vi "Subvi trigger AO DO.vi"(9 "Ext trig enable":bool) -> ()   [LabVIEW 2017]
uses:
  <vilib>/Platform/TimedLoop/XDataNode/timing_clust.ctl
  <vilib>/Platform/TimedLoop/XDataNode/nitl_modes.ctl
  <vilib>/Platform/TimedLoop/XDataNode/wakeup.ctl
  <vilib>/rvi/Emulation/niFpgaSctlEmulationGetInTimedLoop.vi
  <vilib>/rvi/Emulation/niFpgaEmulationReportErrorSimple.vi
  <vilib>/rvi/Emulation/niFpgaGetClockAttributes.vi
  <vilib>/rvi/Emulation/niFpgaCriticalErrorInLSC.vi
  Detector/GV subtrigger.vi
  GV trigger delay.vi
  <vilib>/Platform/TimedLoop/XDataNode/XDataNode.xnode
  <vilib>/Platform/TimedLoop/XDataNode/XDNodeRunTimeDep.lvlib
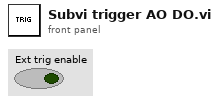
[diagram p1: front panel]
types:
  T1 = typedef "XDNodeRunTimeDep.lvlib/timing_clust.ctl" = cluster{"Expected End [f-1]":u64, "Actual End [f-1]":u64, "Finished Late? [f-1]":bool, "Expected End [i-1]":u64, "Actual End [i-1]":u64, "Finished Late? [i-1]":bool, "Expected Start [i]":u64, "Actual Start [i]":u64, "Expected Start [f]":u64, "Actual Start [f]":u64, "Source Name":string, "Structure Name":string, "Period":i64, "Deadline":i64, "Offset":i64, "Start":i64, "Priority":i32, "Timeout":i32, "Mode":T2, "Wakeup Reason":T3, "Error":errorcluster, "Source Type":string, "Secondary Source Type":string, "Global End Time":u64, "Global Start Time":u64, "Frame Duration":u64, "Iteration Duration":u64, "Assigned CPU":i32, "I/O Scan Engine Mode":u32}
  T2 = typedef "XDNodeRunTimeDep.lvlib/nitl_modes.ctl" = enum32{"No Change", "Process missed periods, maintain original phase", "Discard missed periods, maintain original phase", "Process missed periods, ignore original phase", "Discard missed periods, ignore original phase"}
  T3 = typedef "XDNodeRunTimeDep.lvlib/wakeup.ctl" = enum32{"Normal", "Aborted", "Asynchronous wakeup", "Timing source error", "Timed loop error", "Timeout"}
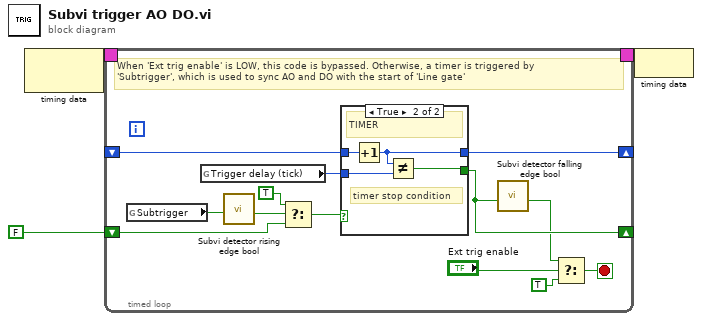
[diagram p0: block diagram]
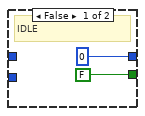
[diagram p2: hidden frame]
diagram:
  n1 = node-c288() -> (w3:T1)  [unwired: 1 in]
  n2 = timed-loop {
    timing: w3 -> [_]
    timing-out: [_] -> w2
    shift-right: [w8] -> _
    shift-left: FALSE -> [w9]
    shift-right: [w12] -> _
    shift-left: _ -> [w11]
    stop <- w6 stop-if-true
    # "When 'Ext trig enable' is LOW, this code is bypassed. Otherwise, a timer is triggered by\n'Subtrigger', which is used to sync AO and DO with the start of 'Line gate'"
    n3 = global read "GV subtrigger.vi" "Subtrigger"() -> (w16:bool)
    n4 = global read "GV trigger delay.vi" "Trigger delay (tick)"() -> (w10:u16)
    n5 = call "Subvi detector rising edge bool.vi"("Input"=w16) -> ("Output"=w13:bool)  [unwired: 10 in]
    n6 = Select(t=TRUE, s=w13, f=w9) -> (s? t:f=w14:bool)
    n7 = case shown="True" w14 {
      tunnel: [FALSE w20] -> w8
      tunnel: [u16 0 w21] -> w12
      tunnel: w11 -> [_ w22]
      tunnel: w10 -> [_ w19]
      frame False {
        # "IDLE"
      }
      frame True {
        # "timer stop condition"
        # "TIMER"
        n8 = Increment(x=w22) -> (x+1=w21:u16)
        n9 = Not Equal?(x=w21, y=w19) -> (x != y?=w20:bool)
      }
    }
    n10 = call "Subvi detector falling edge bool.vi"("Input"=w8) -> ("Output"=w4:bool)  [unwired: 10 in]
    n11 = Select(t=w4, s="Ext trig enable", f=TRUE) -> (s? t:f=w6:bool)
  }
  n12 = node-c288(w2) -> ()
